vi "Update Raw AI.vi"(8 "error in":errorcluster, 11 "AI":T1) -> (0 "error out":errorcluster)   [LabVIEW 2018, in "UDP Writer.lvlib"]
doc: "This subVI enqueues the named action in to the communications queue along with the input data."
uses:
  UDP Writer.lvlib
  Top Level/Shared Controls/Acq Data.ctl
  Private Controls/Module Data.ctl
  Private Controls/Module Action.ctl
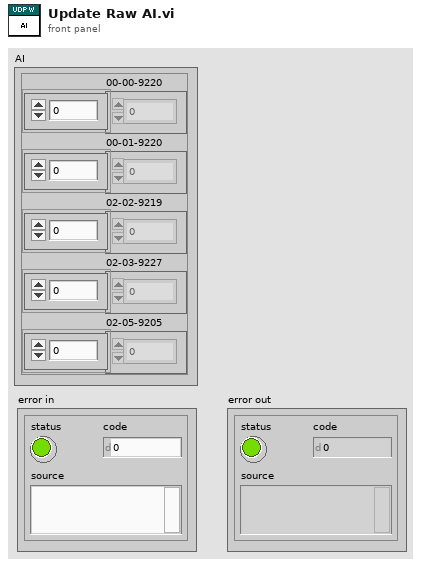
[diagram p1: front panel]
types:
  T1 = typedef "Acq Data.ctl" = cluster{"00-00-9220":dbl[], "00-01-9220":dbl[], "02-02-9219":dbl[], "02-03-9227":dbl[], "02-05-9205":dbl[]}
  T2 = typedef "UDP Writer.lvlib/Module Data.ctl" = cluster{"Data":variant, "Action":T3}
  T3 = typedef "UDP Writer.lvlib/Module Action.ctl" = enum16{"Init", "Update ARINC", "Update Waterfall", "Update RPMs", "Update Temps", "Update Modbus", "Update AI", "Update Vibs", "Write", "Error"}
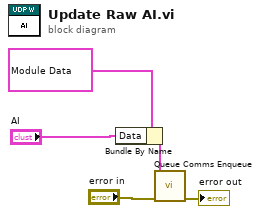
[diagram p0: block diagram]
diagram:
  n1 = Bundle By Name(cluster=T2 {"Data"=variant, "Action"=enum."Update AI"} ("element"), "Data"="AI") -> (w2:T2)
  n2 = call "Queue Comms Enqueue.vi"("error in (no error)"="error in", "element"=w2) -> ("error out"=→"error out":errorcluster)  [unwired: 9 in]
